vi "GlobalSerial.vi"() -> ()   [LabVIEW 2012]
panel:
  out "VISA resource name out":refnum<visa-resource-name>="COM3"
  out "error out":errorcluster
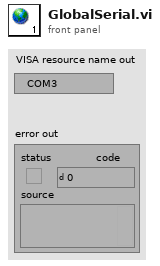
[diagram p1: front panel]
diagram:
